vi "Flush Async.vi"(8 "error in (no error)":errorcluster, 10 "Stop Notifier":refnum<notifier>, 11 "Sift Client In":refnum<class "Sift Client.lvclass">) -> ()   [LabVIEW 2024, in "Sift Stream.lvlib" / "Sift Stream.lvclass"]
uses:
  Sift Stream.lvclass
  <vilib>/Sift/Sift/Sift API/Sift Client.lvclass
  Sift Flush Loop.vi
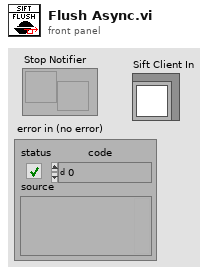
[diagram p1: front panel]
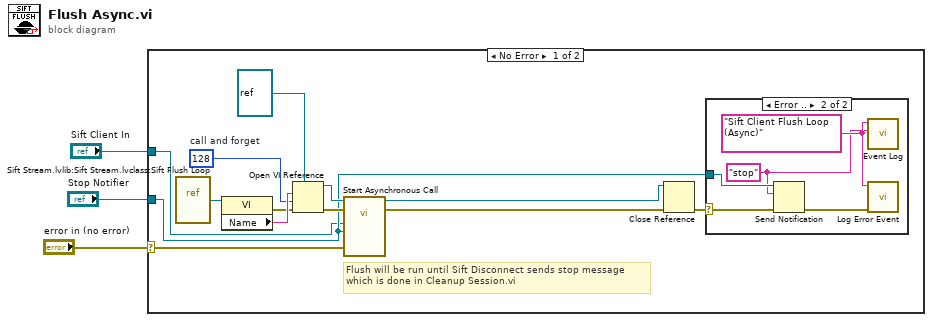
[diagram p0: block diagram]
diagram:
  n1 = case shown="No Error" "error in (no error)" {
    selector: "error in (no error)" -> [w7 _]
    tunnel: "Stop Notifier" -> [w5 _]
    tunnel: "Sift Client In" -> [w4 _]
    frame No Error {
      w8 = 128  # call and forget
      # "Flush will be run until Sift Disconnect sends stop message\nwhich is done in Cleanup Session.vi"
      n2 = vi-ref "Sift Stream.lvlib:Sift Stream.lvclass:Sift Flush Loop.vi"() -> (w12:refnum<vi>)
      n3 = property class="VI"(reference=w12) -> (error out=w10:errorcluster, "Name"=w11:string)  [unwired: 1 in, 1 out]
      n4 = Open VI Reference(type specifier VI Refnum (for type only)=refnum<vi> refnum, vi path=w11, options=w8, error in (no error)=w10) -> (vi reference=w16:refnum<vi>, error out=w15:errorcluster)  [unwired: 2 in]
      n5 = call-by-ref "Start Asynchronous Call"(reference=w16, error in=w15, 8:"error in (no error)"=w7, "Stop Notifier"=w5, "Sift Client In"=w4) -> (reference out=w13:refnum<vi>, error out=w14:errorcluster)  [unwired: 8 in, 1 out]
      n6 = Close Reference(reference=w13, error in (no error)=w14) -> (error out=w6:errorcluster)
      n7 = case shown="Error .." w6 {
        selector: w6 -> [_ w17]
        tunnel: w5 -> [_ w21]
        frame No Error {
        }
        frame Error {
          w20 = "Sift Client Flush Loop (Async)"
          w18 = "stop"
          n8 = Send Notification(notification=w18, notifier=w21, error in (no error)=w17) -> (error out=w19:errorcluster)  [unwired: 1 out]
          n9 = call "Event Log.vi"("Event Type"=w18, "Location"=w20) -> ()  [unwired: 10 in]
          n10 = call "Log Error Event.vi"("error in (no error)"=w19, "Location"=w20) -> ()  [unwired: 10 in]
        }
      }
    }
    frame Error {
    }
  }
